vi "SaveImage_Paper2(SubVI).vi"(7 "RanFilenames":string[](array[string]), 8 "Previous 2":refnum<vi>, 9 "Next 2":refnum<vi>, 10 "connection reference":T1, 11 "Array":refnum<vi>[](array[refnum])) -> ()   [LabVIEW 2013]
uses:
  <vilib>/addons/database/Connection.llb/Conn ObjectReference.ctl
  FYP_LabviewGlobal(SubVI).vi
  <vilib>/addons/database/NI_Database_API.lvlib
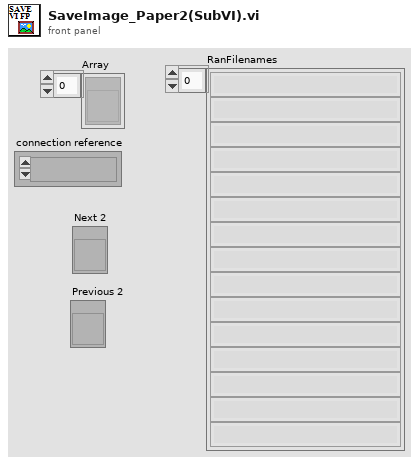
[diagram p1: front panel]
types:
  T1 = typedef "NI_Database_API.lvlib/Conn ObjectReference.ctl" = refnum<k1>
  T2 = typedef "imagedata.ctl" = cluster{"image type":i32, "image depth":i32, "image":u8[], "mask":u8[], "colors":u32[], "Rectangle":cluster{"left":i16, "top":i16, "right":i16, "bottom":i16}}
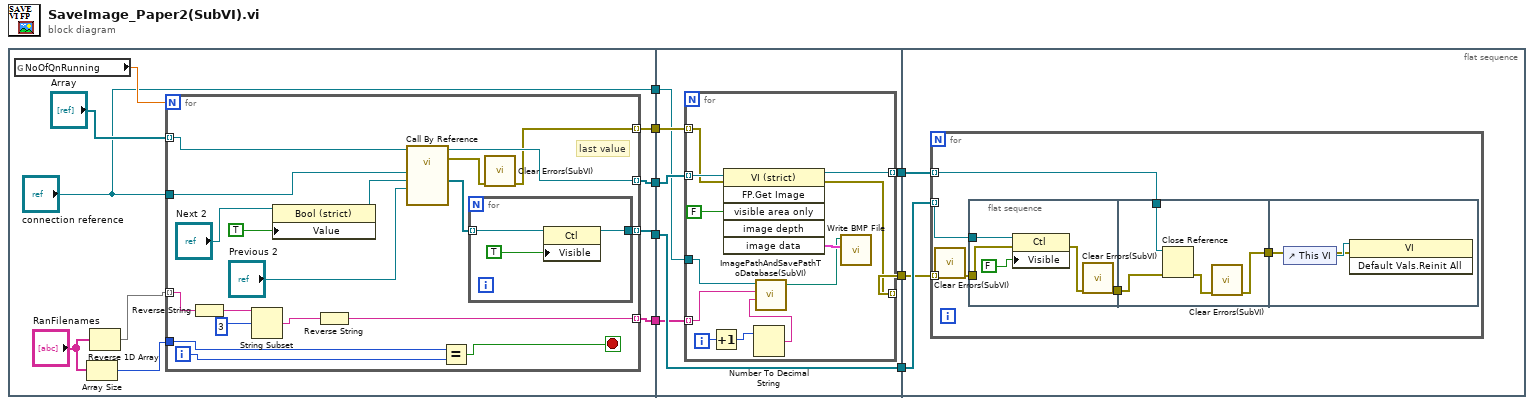
[diagram p0: block diagram]
diagram:
  n1 = flat-sequence {
    tunnel: [w15] -> w8
    tunnel: [w14] -> w7
    tunnel: [w13] -> w6
    tunnel: [w10] -> w3
    tunnel: ["connection reference"] -> w1
    tunnel: w8 -> [w47]
    tunnel: w7 -> [w45]
    tunnel: w6 -> [w46]
    tunnel: [w47] -> w5
    tunnel: [w44] -> w4
    tunnel: w3 -> [w43]
    tunnel: [w42] -> w2
    tunnel: w1 -> [w41]
    tunnel: w5 -> [w61]
    tunnel: w4 -> [w62]
    tunnel: w2 -> [w60]
    frame #0 {
      n2 = global read "FYP_LabviewGlobal(SubVI).vi" "NoOfQnRunning"() -> (w11:dbl)
      n3 = Array Size(array="RanFilenames") -> (size(s)=w12:i32)
      n4 = Reverse 1D Array(array="RanFilenames") -> (reversed array=w17:string[])
      n5 = for {
        N: w11 -> [_]
        tunnel: "Array" -> [w29] mode=indexing
        tunnel: "connection reference" -> [w27]
        tunnel: w17 -> [w35] mode=indexing
        tunnel: [w31] -> w13 mode=indexing
        tunnel: [w28] -> w14 mode=indexing
        tunnel: [w30] -> w15 mode=indexing
        tunnel: w12 -> [w23]
        tunnel: [w19] -> w10 mode=indexing
        i -> [w21]
        stop <- w22 stop-if-true
        # "last value"
        n6 = Reverse String(1:w35) -> (0:w34:string)
        n7 = String Subset(string=w34, offset (0)=3) -> (substring=w33:string)  [unwired: 1 in]
        n8 = property class="Bool (strict)"(reference="Next 2", "Value"=TRUE) -> (reference out=w26:refnum<vi>)  [unwired: 1 in, 1 out]
        n9 = Reverse String(1:w33) -> (0:w31:string)
        n10 = call-by-ref "?"(reference=w29, "Previous 2"="Previous 2", "Next 2"=w26, "connection reference"=w27) -> (reference out=w28:refnum<vi>, error out=w20:errorcluster, "Array"=w24:refnum<vi>[])  [unwired: 9 in]
        n11 = Equal?(x=w23, y=w21) -> (x = y?=w22:bool)
        n12 = for {
          tunnel: w24 -> [w40] mode=indexing
          tunnel: [w38] -> w30
          n13 = property class="Ctl"(reference=w40, "Visible"=TRUE) -> (reference out=w38:refnum<vi>)  [unwired: 1 in, 1 out]
        }
        n14 = call "Clear Errors(SubVI).vi"("error in (no error)"=w20) -> ("error out"=w19:errorcluster)  [unwired: 6 in]
      }
    }
    frame #1 {
      n15 = for {
        tunnel: w46 -> [w51] mode=indexing
        tunnel: w45 -> [w59] mode=indexing
        tunnel: [w58] -> w44 mode=indexing
        tunnel: w43 -> [w55] mode=indexing
        tunnel: [w54] -> w42 mode=indexing
        tunnel: w41 -> [w49]
        i -> [w53]
        n16 = Increment(x=w53) -> (x+1=w52:i32)
        n17 = invoke class="VI (strict)" method="FP.Get Image"(reference=w59, error in=w55, "visible area only"=FALSE ("Visible Area Only")) -> (reference out=w58:refnum<vi>, error out=w54:errorcluster, "image data"=w56:T2)  [unwired: 3 in, 3 out]
        n18 = Number To Decimal String(number=w52) -> (decimal integer string=w48:string)  [unwired: 1 in]
        n19 = call "ImagePathAndSavePathToDatabase(SubVI).vi"("connection reference"=w49, "Name"=w51, "QuestionsNo_Ordered"=w48) -> ("ImagePath"=w50:path)  [unwired: 4 in]
        n20 = call <vilib>:"Write BMP File.vi"("image data"=w56, "path to BMP file"=w50) -> ()  [unwired: 8 in, 2 out]
      }
    }
    frame #2 {
      n21 = for {
        tunnel: w62 -> [w67] mode=indexing
        tunnel: w61 -> [w68] mode=indexing
        tunnel: w60 -> [w66] mode=indexing
        n22 = call "Clear Errors(SubVI).vi"("error in (no error)"=w66) -> ("error out"=w65:errorcluster)  [unwired: 6 in]
        n23 = flat-sequence {
          tunnel: w68 -> [w73]
          tunnel: w65 -> [w71]
          tunnel: [w69] -> w63
          tunnel: w67 -> [w77]
          tunnel: [w74] -> w64
          tunnel: w63 -> [w76]
          tunnel: w64 -> [w78]
          frame #0 {
            n24 = property class="Ctl"(reference=w73, error in=w71, "Visible"=FALSE) -> (error out=w70:errorcluster)  [unwired: 1 out]
            n25 = call "Clear Errors(SubVI).vi"("error in (no error)"=w70) -> ("error out"=w69:errorcluster)  [unwired: 6 in]
          }
          frame #1 {
            n26 = Close Reference(reference=w77, error in (no error)=w76) -> (error out=w75:errorcluster)
            n27 = call "Clear Errors(SubVI).vi"("error in (no error)"=w75) -> ("error out"=w74:errorcluster)  [unwired: 6 in]
          }
          frame #2 {
            n28 = control-ref of="This VI"() -> (w79:refnum<vi>)
            n29 = invoke class="VI" method="Default Vals.Reinit All"(reference=w79, error in=w78) -> ()  [unwired: 1 in, 3 out]
          }
        }
      }
    }
  }
